vi "HandleObservationSync_003.vi"(8 "error in (no error)":errorcluster, 11 "S4GUI in":refnum<class "S4GUI.lvclass">) -> (0 "error out":errorcluster, 3 "S4GUI out":refnum<class "S4GUI.lvclass">)   [LabVIEW 2018, in "S4GUI.lvclass"] (continued)
          n1020 = call-dynamic "Write AcquisitionD.vi"("error in (no error)"=w2625, "Acquisition.lvclass"=w2621, "S4ACS_GUI in"=w2622) -> ("error out"=w2620:errorcluster, "S4ACS_GUI out"=w2619:refnum<class "S4GUI.lvclass">)  [unwired: 7 in]
          n1021 = Compound Arithmetic op=ADD(w2607, w2606, w2605, w2604) -> (w2608:u32)
          n1022 = case shown="0, Default" w2608 {
            tunnel: w2603 -> [w2645 _ _ _ _ _ _ _ _ _ _ _ _ _ _ _]
            tunnel: [w2644 u32 1 ("Obs_state") u32 1 ("Obs_state") u32 1 ("Obs_state") u32 1 ("Obs_state") u32 1 ("Obs_state") u32 1 ("Obs_state") u32 1 ("Obs_state") u32 1 ("Obs_state") u32 1 ("Obs_state") u32 1 ("Obs_state") u32 1 ("Obs_state") u32 1 ("Obs_state") u32 1 ("Obs_state") u32 1 ("Obs_state") u32 1 ("Obs_state")] -> w2609
            tunnel: ["" ("Error Msg") "ERROR: Lost channel 1 connection... - HandleObservationSync.vi state 308" ("Error Msg") "ERROR: Lost channel 2 connection...- HandleObservationSync.vi state 308" ("Error Msg") "ERROR: Lost channels 1 and 2 connection...- HandleObservationSync.vi state 308" ("Error Msg") "ERROR: Lost channel 3 connection...- HandleObservationSync.vi state 308" ("Error Msg") "ERROR: Lost channels 1 and  3 connection...- HandleObservationSync.vi state 308" ("Error Msg") "ERROR:  Lost channels 2 and  3 connection...- HandleObservationSync.vi state 308" ("Error Msg") "ERROR:  Lost channels 1, 2 and  3 connection...- HandleObservationSync.vi state 308" ("Error Msg") "ERROR: Lost channel 4 connection...- HandleObservationSync.vi state 308" ("Error Msg") "ERROR:  Lost channels 1 and 4 connection...- HandleObservationSync.vi state 308" ("Error Msg") "ERROR:  Lost channels 2 and 4 connection...- HandleObservationSync.vi state 308" ("Error Msg") "ERROR: Lost channels 1, 2 and 4 connection...- HandleObservationSync.vi state 308" ("Error Msg") "ERROR: Lost channels 3 and 4 connection...- HandleObservationSync.vi state 308" ("Error Msg") "ERROR: Lost channels 1, 3 and 4 connection...- HandleObservationSync.vi state 308" ("Error Msg") "ERROR: Lost channels 2, 3 and 4 connection...- HandleObservationSync.vi state 308" ("Error Msg") "ERROR: Lost channels 1, 2, 3 and 4 connection...- HandleObservationSync.vi state 308" ("Error Msg")] -> w2610
            frame 0, Default {
              n1023 = Tick Count (ms)() -> (millisecond timer value=w2642:u32)
              n1024 = Increment(x=w2645) -> (x+1=w2644:u32)
              n1025 = local write "time1"(w2642) -> ()
            }
            frame 1 {
            }
            frame 2 {
            }
            frame 3 {
            }
            frame 4 {
            }
            frame 5 {
            }
            frame 6 {
            }
            frame 7 {
            }
            frame 8 {
            }
            frame 9 {
            }
            frame 10 {
            }
            frame 11 {
            }
            frame 12 {
            }
            frame 13 {
            }
            frame 14 {
            }
            frame 15 {
            }
          }
          n1026 = Bundle By Name(cluster=w2619, "Obs_state"=w2609, "Error Msg"=w2610) -> (w2636:refnum<class "S4GUI.lvclass">)
        }
        frame 309 {
          # "Se wait_expose=T, não envia\no EXPOSE do estado 310\n(1o EXPOSE já foi enviado).\n\nNeste caso, vai para:\n* 310 se houver mais \n   de 1 posição da lamina ou para \n* 327 se houver apenas 1 posição\n   da lâmina"
          # "T: mode EXPOSE\nF: mode FIRE"
          # "Espera todos os canais chegarem ao estado ACTIVE\n(estados 54 e 55 de Channel:Run.vi)\n   OU\nTodos os canais incrementarem o Seqs_done. (OV 20240821)"
          n1027 = Unbundle By Name(w2770) -> ("seqAtual"=w2769:u32)
          n1028 = call-dynamic "Read AcquisitionA.vi"("error in (no error)"=w2830, "S4ACS_GUI in"=w2770) -> ("error out"=w2810:errorcluster, "Acquisition.lvclass"=w2811:refnum<class "Acquisition.lvclass">, "S4ACS_GUI out"=w2832:refnum<class "S4GUI.lvclass">)  [unwired: 7 in]
          n1029 = call "Read connection.vi"("error in (no error)"=w2810, "Server in"=w2811) -> ("error out"=w2812:errorcluster, "connection"=w2814:bool, "Server out"=w2813:refnum<class "Acquisition.lvclass">)  [unwired: 7 in]
          n1030 = case shown="True" w2814 {
            tunnel: [w2979 w3003] -> w2833
            tunnel: [w2978 w3002] -> w2831
            tunnel: w2813 -> [w2979 w2995]
            tunnel: w2812 -> [w2978 w2994]
            tunnel: [TRUE w2993] -> w2793
            tunnel: [FALSE w2987] -> w2789
            tunnel: [TRUE w2981] -> w2774
            tunnel: w2769 -> [_ w2980]
            frame False {
            }
            frame True {
              n1031 = call-dynamic "Read Channel.vi"("error in (no error)"=w2994, "Acquisition in"=w2995) -> ("error out"=w2984:errorcluster, "Channel.lvclass"=w2986:refnum<class "Channel.lvclass">, "Acquisition out"=w3004:refnum<class "Acquisition.lvclass">)  [unwired: 7 in]
              n1032 = call-dynamic "Read SequesDone.vi"("error in (no error)"=w2984, "Channel in"=w2986) -> ("error out"=w2983:errorcluster, "SequesDoneRaw"=w2982:u32, "Channel out"=w2985:refnum<class "Channel.lvclass">)  [unwired: 6 in, 1 out]
              n1033 = Equal?(x=w2982, y=w2980) -> (x = y?=w2981:bool)
              n1034 = call-dynamic "Read wait_expose.vi"("error in (no error)"=w2983, "Channel in"=w2985) -> ("error out"=w2988:errorcluster, "wait_expose"=w2987:bool, "Channel out"=w2989:refnum<class "Channel.lvclass">)  [unwired: 7 in]
              n1035 = call-dynamic "Read State Machine.vi"("error in (no error)"=w2988, "Device in"=w2989) -> ("error out"=w2996:errorcluster, "State Machine.lvclass"=w2998:refnum<class "State Machine.lvclass">, "Device out"=w3000:refnum<class "Channel.lvclass">)  [unwired: 7 in]
              n1036 = call-dynamic "Read State.vi"("error in (no error)"=w2996, "State Machine in"=w2998) -> ("error out"=w2990:errorcluster, "State"=w2992:i32, "State Machine out"=w2997:refnum<class "State Machine.lvclass">)  [unwired: 7 in]
              n1037 = Greater?(x=w2992, y=53) -> (0:w2993:bool)
              n1038 = call-dynamic "Write State Machine.vi"("error in (no error)"=w2990, "State Machine.lvclass"=w2997, "Device in"=w3000) -> ("error out"=w2999:errorcluster, "Device out"=w3001:refnum<class "Channel.lvclass">)  [unwired: 7 in]
              n1039 = call-dynamic "Write Channel.vi"("error in (no error)"=w2999, "Channel.lvclass"=w3001, "Acquisition in"=w3004) -> ("error out"=w3002:errorcluster, "Acquisition out"=w3003:refnum<class "Acquisition.lvclass">)  [unwired: 7 in]
            }
          }
          n1040 = call-dynamic "Write AcquisitionA.vi"("error in (no error)"=w2831, "Acquisition.lvclass"=w2833, "S4ACS_GUI in"=w2832) -> ("error out"=w2827:errorcluster, "S4ACS_GUI out"=w2828:refnum<class "S4GUI.lvclass">)  [unwired: 7 in]
          n1041 = call "Read AcquisitionB.vi"("error in (no error)"=w2827, "S4ACS_GUI in"=w2828) -> ("error out"=w2807:errorcluster, "Acquisition.lvclass"=w2809:refnum<class "Acquisition.lvclass">, "S4ACS_GUI out"=w2825:refnum<class "S4GUI.lvclass">)  [unwired: 7 in]
          n1042 = call "Read connection.vi"("error in (no error)"=w2807, "Server in"=w2809) -> ("error out"=w2806:errorcluster, "connection"=w2805:bool, "Server out"=w2808:refnum<class "Acquisition.lvclass">)  [unwired: 7 in]
          n1043 = case shown="True" w2805 {
            tunnel: w2808 -> [w2949 w2974]
            tunnel: w2806 -> [w2948 w2973]
            tunnel: [w2949 w2971] -> w2826
            tunnel: [w2948 w2970] -> w2824
            tunnel: [TRUE w2961] -> w2792
            tunnel: [FALSE ("expose") w2957] -> w2788
            tunnel: [TRUE w2951] -> w2776
            tunnel: w2769 -> [_ w2950]
            frame False {
            }
            frame True {
              n1044 = call-dynamic "Read Channel.vi"("error in (no error)"=w2973, "Acquisition in"=w2974) -> ("error out"=w2953:errorcluster, "Channel.lvclass"=w2956:refnum<class "Channel.lvclass">, "Acquisition out"=w2972:refnum<class "Acquisition.lvclass">)  [unwired: 7 in]
              n1045 = call-dynamic "Read SequesDone.vi"("error in (no error)"=w2953, "Channel in"=w2956) -> ("error out"=w2952:errorcluster, "SequesDoneRaw"=w2954:u32, "Channel out"=w2955:refnum<class "Channel.lvclass">)  [unwired: 6 in, 1 out]
              n1046 = Equal?(x=w2954, y=w2950) -> (x = y?=w2951:bool)
              n1047 = call-dynamic "Read wait_expose.vi"("error in (no error)"=w2952, "Channel in"=w2955) -> ("error out"=w2958:errorcluster, "wait_expose"=w2957:bool, "Channel out"=w2959:refnum<class "Channel.lvclass">)  [unwired: 7 in]
              n1048 = call-dynamic "Read State Machine.vi"("error in (no error)"=w2958, "Device in"=w2959) -> ("error out"=w2964:errorcluster, "State Machine.lvclass"=w2966:refnum<class "State Machine.lvclass">, "Device out"=w2968:refnum<class "Channel.lvclass">)  [unwired: 7 in]
              n1049 = call-dynamic "Read State.vi"("error in (no error)"=w2964, "State Machine in"=w2966) -> ("error out"=w2963:errorcluster, "State"=w2960:i32, "State Machine out"=w2965:refnum<class "State Machine.lvclass">)  [unwired: 7 in]
              n1050 = Greater?(x=w2960, y=53) -> (0:w2961:bool)
              n1051 = call-dynamic "Write State Machine.vi"("error in (no error)"=w2963, "State Machine.lvclass"=w2965, "Device in"=w2968) -> ("error out"=w2967:errorcluster, "Device out"=w2969:refnum<class "Channel.lvclass">)  [unwired: 7 in]
              n1052 = call-dynamic "Write Channel.vi"("error in (no error)"=w2967, "Channel.lvclass"=w2969, "Acquisition in"=w2972) -> ("error out"=w2970:errorcluster, "Acquisition out"=w2971:refnum<class "Acquisition.lvclass">)  [unwired: 7 in]
            }
          }
          n1053 = call "Write AcquisitionB.vi"("error in (no error)"=w2824, "Acquisition.lvclass"=w2826, "S4ACS_GUI in"=w2825) -> ("error out"=w2820:errorcluster, "S4ACS_GUI out"=w2819:refnum<class "S4GUI.lvclass">)  [unwired: 7 in]
          n1054 = call-dynamic "Read AcquisitionC.vi"("error in (no error)"=w2820, "S4ACS_GUI in"=w2819) -> ("error out"=w2802:errorcluster, "Acquisition.lvclass"=w2804:refnum<class "Acquisition.lvclass">, "S4ACS_GUI out"=w2822:refnum<class "S4GUI.lvclass">)  [unwired: 7 in]
          n1055 = call "Read connection.vi"("error in (no error)"=w2802, "Server in"=w2804) -> ("error out"=w2801:errorcluster, "connection"=w2800:bool, "Server out"=w2803:refnum<class "Acquisition.lvclass">)  [unwired: 7 in]
          n1056 = case shown="True" w2800 {
            tunnel: [w2918 w2939] -> w2823
            tunnel: [w2919 w2938] -> w2821
            tunnel: w2803 -> [w2919 w2934]
            tunnel: w2801 -> [w2918 w2933]
            tunnel: [TRUE w2930] -> w2791
            tunnel: [FALSE ("expose") w2927] -> w2787
            tunnel: [TRUE w2921] -> w2775
            tunnel: w2769 -> [_ w2920]
            frame False {
            }
            frame True {
              n1057 = call-dynamic "Read Channel.vi"("error in (no error)"=w2933, "Acquisition in"=w2934) -> ("error out"=w2926:errorcluster, "Channel.lvclass"=w2925:refnum<class "Channel.lvclass">, "Acquisition out"=w2937:refnum<class "Acquisition.lvclass">)  [unwired: 7 in]
              n1058 = call-dynamic "Read SequesDone.vi"("error in (no error)"=w2926, "Channel in"=w2925) -> ("error out"=w2922:errorcluster, "SequesDoneRaw"=w2923:u32, "Channel out"=w2924:refnum<class "Channel.lvclass">)  [unwired: 6 in, 1 out]
              n1059 = Equal?(x=w2923, y=w2920) -> (x = y?=w2921:bool)
              n1060 = call-dynamic "Read wait_expose.vi"("error in (no error)"=w2922, "Channel in"=w2924) -> ("error out"=w2928:errorcluster, "wait_expose"=w2927:bool, "Channel out"=w2929:refnum<class "Channel.lvclass">)  [unwired: 7 in]
              n1061 = call-dynamic "Read State Machine.vi"("error in (no error)"=w2928, "Device in"=w2929) -> ("error out"=w2935:errorcluster, "State Machine.lvclass"=w2943:refnum<class "State Machine.lvclass">, "Device out"=w2941:refnum<class "Channel.lvclass">)  [unwired: 7 in]
              n1062 = call-dynamic "Read State.vi"("error in (no error)"=w2935, "State Machine in"=w2943) -> ("error out"=w2936:errorcluster, "State"=w2931:i32, "State Machine out"=w2944:refnum<class "State Machine.lvclass">)  [unwired: 7 in]
              n1063 = Greater?(x=w2931, y=53) -> (0:w2930:bool)
              n1064 = call-dynamic "Write State Machine.vi"("error in (no error)"=w2936, "State Machine.lvclass"=w2944, "Device in"=w2941) -> ("error out"=w2942:errorcluster, "Device out"=w2940:refnum<class "Channel.lvclass">)  [unwired: 7 in]
              n1065 = call-dynamic "Write Channel.vi"("error in (no error)"=w2942, "Channel.lvclass"=w2940, "Acquisition in"=w2937) -> ("error out"=w2939:errorcluster, "Acquisition out"=w2938:refnum<class "Acquisition.lvclass">)  [unwired: 7 in]
            }
          }
          n1066 = call-dynamic "Write AcquisitionC.vi"("error in (no error)"=w2823, "Acquisition.lvclass"=w2821, "S4ACS_GUI in"=w2822) -> ("error out"=w2799:errorcluster, "S4ACS_GUI out"=w2815:refnum<class "S4GUI.lvclass">)  [unwired: 7 in]
          n1067 = call-dynamic "Read AcquisitionD.vi"("error in (no error)"=w2799, "S4ACS_GUI in"=w2815) -> ("error out"=w2795:errorcluster, "Acquisition.lvclass"=w2798:refnum<class "Acquisition.lvclass">, "S4ACS_GUI out"=w2817:refnum<class "S4GUI.lvclass">)  [unwired: 7 in]
          n1068 = call "Read connection.vi"("error in (no error)"=w2795, "Server in"=w2798) -> ("error out"=w2796:errorcluster, "connection"=w2794:bool, "Server out"=w2797:refnum<class "Acquisition.lvclass">)  [unwired: 7 in]
          n1069 = case shown="True" w2794 {
            tunnel: [w2889 w2913] -> w2818
            tunnel: [w2888 w2912] -> w2816
            tunnel: [TRUE w2901] -> w2790
            tunnel: w2797 -> [w2889 w2904]
            tunnel: w2796 -> [w2888 w2903]
            tunnel: [FALSE ("expose") w2897] -> w2786
            tunnel: [TRUE w2891] -> w2777
            tunnel: w2769 -> [_ w2890]
            frame False {
            }
            frame True {
              n1070 = call-dynamic "Read Channel.vi"("error in (no error)"=w2903, "Acquisition in"=w2904) -> ("error out"=w2895:errorcluster, "Channel.lvclass"=w2896:refnum<class "Channel.lvclass">, "Acquisition out"=w2914:refnum<class "Acquisition.lvclass">)  [unwired: 7 in]
              n1071 = call-dynamic "Read SequesDone.vi"("error in (no error)"=w2895, "Channel in"=w2896) -> ("error out"=w2893:errorcluster, "SequesDoneRaw"=w2894:u32, "Channel out"=w2892:refnum<class "Channel.lvclass">)  [unwired: 6 in, 1 out]
              n1072 = Equal?(x=w2894, y=w2890) -> (x = y?=w2891:bool)
              n1073 = call-dynamic "Read wait_expose.vi"("error in (no error)"=w2893, "Channel in"=w2892) -> ("error out"=w2898:errorcluster, "wait_expose"=w2897:bool, "Channel out"=w2899:refnum<class "Channel.lvclass">)  [unwired: 7 in]
              n1074 = call-dynamic "Read State Machine.vi"("error in (no error)"=w2898, "Device in"=w2899) -> ("error out"=w2906:errorcluster, "State Machine.lvclass"=w2908:refnum<class "State Machine.lvclass">, "Device out"=w2910:refnum<class "Channel.lvclass">)  [unwired: 7 in]
              n1075 = call-dynamic "Read State.vi"("error in (no error)"=w2906, "State Machine in"=w2908) -> ("error out"=w2905:errorcluster, "State"=w2900:i32, "State Machine out"=w2907:refnum<class "State Machine.lvclass">)  [unwired: 7 in]
              n1076 = Greater?(x=w2900, y=53) -> (0:w2901:bool)
              n1077 = call-dynamic "Write State Machine.vi"("error in (no error)"=w2905, "State Machine.lvclass"=w2907, "Device in"=w2910) -> ("error out"=w2909:errorcluster, "Device out"=w2911:refnum<class "Channel.lvclass">)  [unwired: 7 in]
              n1078 = call-dynamic "Write Channel.vi"("error in (no error)"=w2909, "Channel.lvclass"=w2911, "Acquisition in"=w2914) -> ("error out"=w2912:errorcluster, "Acquisition out"=w2913:refnum<class "Acquisition.lvclass">)  [unwired: 7 in]
            }
          }
          n1079 = call-dynamic "Write AcquisitionD.vi"("error in (no error)"=w2816, "Acquisition.lvclass"=w2818, "S4ACS_GUI in"=w2817) -> ("error out"=w2768:errorcluster, "S4ACS_GUI out"=w2766:refnum<class "S4GUI.lvclass">)  [unwired: 7 in]
          n1080 = Compound Arithmetic op=OR(w2789, w2788, w2787, w2786) -> (w2779:bool)
          n1081 = Compound Arithmetic op=AND(w2774, w2776, w2775, w2777) -> (w2772:bool)
          n1082 = Compound Arithmetic op=AND(w2793, w2792, w2791, w2790) -> (w2773:bool)
          n1083 = Or(x=w2773, y=w2772) -> (x .or. y?=w2771:bool)
          n1084 = call-dynamic "VerifErrors.vi"("error in (no error)"=w2768, "S4GUI in"=w2766) -> ("error out"=w2767:errorcluster, "Error value"=w2764:u32, "S4GUI out"=w2765:refnum<class "S4GUI.lvclass">)  [unwired: 7 in]
          n1085 = call-dynamic "VerifWavePlate.vi"("error in (no error)"=w2767, "S4GUI in"=w2765) -> ("error out"=w2783:errorcluster, "One Position"=w2785:bool, "S4GUI out"=w2784:refnum<class "S4GUI.lvclass">)  [unwired: 7 in]
          n1086 = case shown="True" w2785 {
            tunnel: w2784 -> [w2866 w2883]
            tunnel: [u32 312 ("t") u32 327 ("t")] -> w2781
            tunnel: [w2866 w2869] -> w2780
            tunnel: w2783 -> [w2864 w2868]
            tunnel: [w2864 w2867] -> w2782
            frame False {
            }
            frame True {
              # "Recarrega SEQ, antes de desviar\n para tratamento de fotometria."
              n1087 = call "Read Instrument.lvclass.vi"("error in (no error)"=w2868, "S4ACS_GUI in"=w2883) -> ("error out"=w2878:errorcluster, "Instrument.lvclass"=w2882:refnum<class "Instrument.lvclass">, "S4ACS_GUI out"=w2881:refnum<class "S4GUI.lvclass">)  [unwired: 7 in]
              n1088 = call "Read WPROT.vi"("error in (no error)"=w2878, "Instrument in"=w2882) -> ("error out"=w2871:errorcluster, "Opt_Selector.lvclass"=w2874:refnum<class "Opt_Selector.lvclass">, "Instrument out"=w2879:refnum<class "Instrument.lvclass">)  [unwired: 7 in]
              n1089 = call-dynamic "Read sequencia_ant.vi"("error in (no error)"=w2871, "Opt_Selector in"=w2874) -> ("error out"=w2876:errorcluster, "sequencia_ant"=w2875:u16, "Opt_Selector out"=w2873:refnum<class "Opt_Selector.lvclass">)  [unwired: 7 in]
              n1090 = call-dynamic "Write sequencia.vi"("error in (no error)"=w2876, "sequencia"=w2875, "Opt_Selector in"=w2873) -> ("error out"=w2870:errorcluster, "Opt_Selector out"=w2872:refnum<class "Opt_Selector.lvclass">)  [unwired: 7 in]
              n1091 = call "Write WPROT.vi"("error in (no error)"=w2870, "Opt_Selector.lvclass"=w2872, "Instrument in"=w2879) -> ("error out"=w2877:errorcluster, "Instrument out"=w2880:refnum<class "Instrument.lvclass">)  [unwired: 7 in]
              n1092 = call "Write Instrument.lvclass.vi"("error in (no error)"=w2877, "Instrument.lvclass"=w2880, "S4ACS_GUI in"=w2881) -> ("error out"=w2867:errorcluster, "S4ACS_GUI out"=w2869:refnum<class "S4GUI.lvclass">)  [unwired: 7 in]
            }
          }
          n1093 = case shown="False" w2771 {
            tunnel: w2780 -> [w2836 w2863]
            tunnel: [w2842 w2862] -> w2778
            tunnel: w2781 -> [_ w2860]
            tunnel: w2764 -> [w2834 _]
            frame False {
              # "Aguardando iniciar exposição por 5s"
              n1094 = Tick Count (ms)() -> (millisecond timer value=w2841:u32)
              n1095 = local read "time1"() -> (w2835:u32)
              n1096 = Subtract(x=w2841, y=w2835) -> (x-y=w2838:u32)
              n1097 = To Double Precision Float(number=w2838) -> (double precision float=w2840:dbl)
              n1098 = Less?(x=5000.0 ("y"), y=w2840) -> (x < y?=w2839:bool)
              n1099 = case shown="False" w2839 {
                tunnel: w2836 -> [w2844 w2858]
                tunnel: [w2843 w2857] -> w2842
                tunnel: w2834 -> [w2845 _]
                frame False {
                  n1100 = case shown="1..15" w2845 {
                    selector: w2845 -> [_ w2853]
                    tunnel: [w2846 w2848] -> w2843
                    tunnel: w2844 -> [w2846 w2854]
                    frame 0, Default {
                    }
                    frame 1..15 {
                      n1101 = Number To Decimal String(number=w2853) -> (decimal integer string=w2850:string)  [unwired: 1 in]
                      n1102 = Concatenate Strings("CHANNEL ERROR <", w2850, ">: Error flag TRUE - see ACS panel.  HandleObservationSync.vi - state 309.") -> (w2852:string)
                      n1103 = Bundle By Name(cluster=w2854, "Obs_state"=u32 1, "Error Msg"=w2852) -> (w2848:refnum<class "S4GUI.lvclass">)
                    }
                  }
                }
                frame True {
                  n1104 = Bundle By Name(cluster=w2858, "Obs_state"=u32 1, "Error Msg"="ERROR: Acquisition Timeout. HandleObservationSync.vi - state 309.") -> (w2857:refnum<class "S4GUI.lvclass">)
                }
              }
            }
            frame True {
              # "Iniciou aquisição..."
              n1105 = Tick Count (ms)() -> (millisecond timer value=→"time308":u32)
              n1106 = Tick Count (ms)() -> (millisecond timer value=w2861:u32)
              n1107 = Bundle By Name(cluster=w2863, "Obs_state"=w2860) -> (w2862:refnum<class "S4GUI.lvclass">)
              n1108 = local write "time307"(w2861) -> ()
              n1109 = local write "time1"(w2861) -> ()
            }
          }
          n1110 = Bundle By Name(cluster=w2778, "mode EXPOSE"=w2779) -> (w2829:refnum<class "S4GUI.lvclass">)
        }
        frame 312 {
          # "Verifcando avanço de SEQUENCIA:"
          # "T=canais receberam STOP"
          # "T= Todos os canais ativos na mesma sequencia;\nF= Canais com sequencia diferente"
          # "Todos os SEQ_DONE \nsão iguais a SeqAtual?\nSe sim, avança lâmina."
          # "Exemplo:\nSET #CYCLES 3\nSET #SEQ 4\ntotal de sequencias: 3 x 4 = 12\n\nseq.        CYCLES_DONE           SEQS_DONE\n1a.                     0                                 0\n2a.                     0                                 1 \n3a.                     0                                 2 \n4a.                     0                                 3 \n                          1                                 4\n5a.                     1                                 0 \n6a.                     1                                 1 \n7a.                     1                                 2 \n8a.                     1                                 3 \n                          2                                 4\n9a.                     2                                 0 \n10a.                   2                                 1 \n11a.                   2                                 2 \n12a.                   2                                 3 \n\nfim                    3                                 4"
          n1111 = Unbundle By Name(w3030) -> ("seqAtual"=w3027:u32)
          n1112 = call-dynamic "Read AcquisitionA.vi"("error in (no error)"=w3064, "S4ACS_GUI in"=w3030) -> ("error out"=w3045:errorcluster, "Acquisition.lvclass"=w3046:refnum<class "Acquisition.lvclass">, "S4ACS_GUI out"=w3066:refnum<class "S4GUI.lvclass">)  [unwired: 7 in]
          n1113 = call-dynamic "Read enabled.vi"("error in (no error)"=w3045, "Server in"=w3046) -> ("error out"=w3044:errorcluster, "enabled"=w3019:bool, "Server out"=w3043:refnum<class "Acquisition.lvclass">)  [unwired: 7 in]
          n1114 = case shown="True" w3019 {
            tunnel: w3044 -> [w3215 w3231]
            tunnel: [w3216 w3229] -> w3067
            tunnel: [w3215 w3228] -> w3065
            tunnel: [u32 0 ("SequesDone") w3217] -> w3024
            tunnel: w3043 -> [w3216 w3227]
            tunnel: w3027 -> [_ w3226]
            tunnel: [TRUE w3225] -> w3029
            tunnel: [FALSE ("stopping") w3218] -> w3012
            frame False {
            }
            frame True {
              # "SEQS_DONE = 0,1,2,...,n,0,1,..."
              n1115 = call-dynamic "Read Channel.vi"("error in (no error)"=w3231, "Acquisition in"=w3227) -> ("error out"=w3223:errorcluster, "Channel.lvclass"=w3224:refnum<class "Channel.lvclass">, "Acquisition out"=w3230:refnum<class "Acquisition.lvclass">)  [unwired: 7 in]
              n1116 = call-dynamic "Read SequesDone.vi"("error in (no error)"=w3223, "Channel in"=w3224) -> ("error out"=w3221:errorcluster, "SequesDoneRaw"=w3217:u32, "Channel out"=w3222:refnum<class "Channel.lvclass">)  [unwired: 6 in, 1 out]
              n1117 = Equal?(x=w3217, y=w3226) -> (x = y?=w3225:bool)
              n1118 = call-dynamic "Read stopping.vi"("error in (no error)"=w3221, "Channel in"=w3222) -> ("error out"=w3220:errorcluster, "stopping"=w3218:bool, "Channel out"=w3219:refnum<class "Channel.lvclass">)  [unwired: 7 in]
              n1119 = call-dynamic "Write Channel.vi"("error in (no error)"=w3220, "Channel.lvclass"=w3219, "Acquisition in"=w3230) -> ("error out"=w3228:errorcluster, "Acquisition out"=w3229:refnum<class "Acquisition.lvclass">)  [unwired: 7 in]
            }
          }
          n1120 = call-dynamic "Write AcquisitionA.vi"("error in (no error)"=w3065, "Acquisition.lvclass"=w3067, "S4ACS_GUI in"=w3066) -> ("error out"=w3062:errorcluster, "S4ACS_GUI out"=w3061:refnum<class "S4GUI.lvclass">)  [unwired: 7 in]
          n1121 = call "Read AcquisitionB.vi"("error in (no error)"=w3062, "S4ACS_GUI in"=w3061) -> ("error out"=w3039:errorcluster, "Acquisition.lvclass"=w3042:refnum<class "Acquisition.lvclass">, "S4ACS_GUI out"=w3063:refnum<class "S4GUI.lvclass">)  [unwired: 7 in]
          n1122 = call-dynamic "Read enabled.vi"("error in (no error)"=w3039, "Server in"=w3042) -> ("error out"=w3040:errorcluster, "enabled"=w3018:bool, "Server out"=w3041:refnum<class "Acquisition.lvclass">)  [unwired: 7 in]
          n1123 = case shown="True" w3018 {
            tunnel: w3040 -> [w3195 w3211]
            tunnel: w3041 -> [w3196 w3210]
            tunnel: [u32 0 ("SequesDone") w3197] -> w3021
            tunnel: [w3195 w3209] -> w3060
            tunnel: [w3196 w3208] -> w3059
            tunnel: w3027 -> [_ w3205]
            tunnel: [TRUE w3204] -> w3028
            tunnel: [FALSE ("stopping") w3198] -> w3011
            frame False {
            }
            frame True {
              n1124 = call-dynamic "Read Channel.vi"("error in (no error)"=w3211, "Acquisition in"=w3210) -> ("error out"=w3202:errorcluster, "Channel.lvclass"=w3203:refnum<class "Channel.lvclass">, "Acquisition out"=w3206:refnum<class "Acquisition.lvclass">)  [unwired: 7 in]
              n1125 = call-dynamic "Read SequesDone.vi"("error in (no error)"=w3202, "Channel in"=w3203) -> ("error out"=w3200:errorcluster, "SequesDoneRaw"=w3197:u32, "Channel out"=w3207:refnum<class "Channel.lvclass">)  [unwired: 6 in, 1 out]
              n1126 = Equal?(x=w3197, y=w3205) -> (x = y?=w3204:bool)
              n1127 = call-dynamic "Read stopping.vi"("error in (no error)"=w3200, "Channel in"=w3207) -> ("error out"=w3199:errorcluster, "stopping"=w3198:bool, "Channel out"=w3201:refnum<class "Channel.lvclass">)  [unwired: 7 in]
              n1128 = call-dynamic "Write Channel.vi"("error in (no error)"=w3199, "Channel.lvclass"=w3201, "Acquisition in"=w3206) -> ("error out"=w3209:errorcluster, "Acquisition out"=w3208:refnum<class "Acquisition.lvclass">)  [unwired: 7 in]
            }
          }
          n1129 = call "Write AcquisitionB.vi"("error in (no error)"=w3060, "Acquisition.lvclass"=w3059, "S4ACS_GUI in"=w3063) -> ("error out"=w3052:errorcluster, "S4ACS_GUI out"=w3051:refnum<class "S4GUI.lvclass">)  [unwired: 7 in]
          n1130 = call-dynamic "Read AcquisitionC.vi"("error in (no error)"=w3052, "S4ACS_GUI in"=w3051) -> ("error out"=w3036:errorcluster, "Acquisition.lvclass"=w3038:refnum<class "Acquisition.lvclass">, "S4ACS_GUI out"=w3054:refnum<class "S4GUI.lvclass">)  [unwired: 7 in]
          n1131 = call-dynamic "Read enabled.vi"("error in (no error)"=w3036, "Server in"=w3038) -> ("error out"=w3035:errorcluster, "enabled"=w3017:bool, "Server out"=w3037:refnum<class "Acquisition.lvclass">)  [unwired: 7 in]
          n1132 = case shown="True" w3017 {
            tunnel: [w3175 w3191] -> w3055
            tunnel: [w3176 w3190] -> w3053
            tunnel: w3035 -> [w3175 w3187]
            tunnel: w3037 -> [w3176 w3188]
            tunnel: [u32 0 ("SequesDone") w3177] -> w3020
            tunnel: w3027 -> [_ w3186]
            tunnel: [TRUE w3185] -> w3026
            tunnel: [FALSE ("stopping") w3178] -> w3010
            frame False {
            }
            frame True {
              n1133 = call-dynamic "Read Channel.vi"("error in (no error)"=w3187, "Acquisition in"=w3188) -> ("error out"=w3182:errorcluster, "Channel.lvclass"=w3183:refnum<class "Channel.lvclass">, "Acquisition out"=w3189:refnum<class "Acquisition.lvclass">)  [unwired: 7 in]
              n1134 = call-dynamic "Read SequesDone.vi"("error in (no error)"=w3182, "Channel in"=w3183) -> ("error out"=w3180:errorcluster, "SequesDoneRaw"=w3177:u32, "Channel out"=w3184:refnum<class "Channel.lvclass">)  [unwired: 6 in, 1 out]
              n1135 = Equal?(x=w3177, y=w3186) -> (x = y?=w3185:bool)
              n1136 = call-dynamic "Read stopping.vi"("error in (no error)"=w3180, "Channel in"=w3184) -> ("error out"=w3179:errorcluster, "stopping"=w3178:bool, "Channel out"=w3181:refnum<class "Channel.lvclass">)  [unwired: 7 in]
              n1137 = call-dynamic "Write Channel.vi"("error in (no error)"=w3179, "Channel.lvclass"=w3181, "Acquisition in"=w3189) -> ("error out"=w3191:errorcluster, "Acquisition out"=w3190:refnum<class "Acquisition.lvclass">)  [unwired: 7 in]
            }
          }
          n1138 = call-dynamic "Write AcquisitionC.vi"("error in (no error)"=w3055, "Acquisition.lvclass"=w3053, "S4ACS_GUI in"=w3054) -> ("error out"=w3049:errorcluster, "S4ACS_GUI out"=w3050:refnum<class "S4GUI.lvclass">)  [unwired: 7 in]
          n1139 = call-dynamic "Read AcquisitionD.vi"("error in (no error)"=w3049, "S4ACS_GUI in"=w3050) -> ("error out"=w3032:errorcluster, "Acquisition.lvclass"=w3034:refnum<class "Acquisition.lvclass">, "S4ACS_GUI out"=w3056:refnum<class "S4GUI.lvclass">)  [unwired: 7 in]
          n1140 = call-dynamic "Read enabled.vi"("error in (no error)"=w3032, "Server in"=w3034) -> ("error out"=w3031:errorcluster, "enabled"=w3016:bool, "Server out"=w3033:refnum<class "Acquisition.lvclass">)  [unwired: 7 in]
          n1141 = Build Array(w3019, w3018, w3017, w3016) -> (w3015:bool[])
          n1142 = case shown="True" w3016 {
            tunnel: [w3156 w3171] -> w3058
            tunnel: [w3155 w3170] -> w3057
            tunnel: w3033 -> [w3156 w3169]
            tunnel: w3031 -> [w3155 w3168]
            tunnel: [u32 0 ("SequesDone") w3157] -> w3023
            tunnel: w3027 -> [_ w3166]
            tunnel: [TRUE w3165] -> w3025
            tunnel: [FALSE ("stopping") w3158] -> w3009
            frame False {
            }
            frame True {
              n1143 = call-dynamic "Read Channel.vi"("error in (no error)"=w3168, "Acquisition in"=w3169) -> ("error out"=w3162:errorcluster, "Channel.lvclass"=w3163:refnum<class "Channel.lvclass">, "Acquisition out"=w3167:refnum<class "Acquisition.lvclass">)  [unwired: 7 in]
              n1144 = call-dynamic "Read SequesDone.vi"("error in (no error)"=w3162, "Channel in"=w3163) -> ("error out"=w3160:errorcluster, "SequesDoneRaw"=w3157:u32, "Channel out"=w3164:refnum<class "Channel.lvclass">)  [unwired: 6 in, 1 out]
              n1145 = Equal?(x=w3157, y=w3166) -> (x = y?=w3165:bool)
              n1146 = call-dynamic "Read stopping.vi"("error in (no error)"=w3160, "Channel in"=w3164) -> ("error out"=w3159:errorcluster, "stopping"=w3158:bool, "Channel out"=w3161:refnum<class "Channel.lvclass">)  [unwired: 7 in]
              n1147 = call-dynamic "Write Channel.vi"("error in (no error)"=w3159, "Channel.lvclass"=w3161, "Acquisition in"=w3167) -> ("error out"=w3170:errorcluster, "Acquisition out"=w3171:refnum<class "Acquisition.lvclass">)  [unwired: 7 in]
            }
          }
          n1148 = Boolean Array To Number(Boolean array=w3015) -> (number=w3013:u32)
          n1149 = Compound Arithmetic op=AND(w3029, w3028, w3026, w3025) -> (w3014:bool)
          n1150 = Compound Arithmetic op=OR(w3012, w3011, w3010, w3009) -> (w3008:bool)
          n1151 = case shown="11" w3013 {
            tunnel: w3024 -> [w3075 _ w3087 _ w3096 _ w3102 w3108 _ w3114 w3117 _]
            tunnel: w3023 -> [w3074 w3078 w3083 w3090 w3091 w3099 w3101 _ _ _ _ _]
            tunnel: w3021 -> [w3073 w3076 _ _ w3095 w3097 _ w3107 w3111 _ w3116 _]
            tunnel: w3020 -> [w3072 w3077 w3082 w3088 _ _ _ w3106 w3110 w3113 _ _]
            tunnel: [w3068 w3079 w3084 w3089 w3092 w3098 w3100 w3103 w3109 w3112 w3115 TRUE] -> _
            frame 15 {
              # "A,B,C,D ativos"
              n1152 = Equal?(x=w3075, y=w3073) -> (x = y?=w3071:bool)
              n1153 = Equal?(x=w3072, y=w3074) -> (x = y?=w3069:bool)
              n1154 = Equal?(x=w3073, y=w3072) -> (x = y?=w3070:bool)
              n1155 = Compound Arithmetic op=AND(w3071, w3070, w3069) -> (w3068:bool)
            }
            frame 14 {
              # "B,C e,D ativos"
              n1156 = Equal?(x=w3076, y=w3077) -> (x = y?=w3081:bool)
              n1157 = Equal?(x=w3077, y=w3078) -> (x = y?=w3080:bool)
              n1158 = Compound Arithmetic op=AND(w3081, w3080) -> (w3079:bool)
            }
            frame 13 {
              # "A,C e,D ativos"
              n1159 = Equal?(x=w3087, y=w3082) -> (x = y?=w3086:bool)
              n1160 = Equal?(x=w3082, y=w3083) -> (x = y?=w3085:bool)
              n1161 = Compound Arithmetic op=AND(w3086, w3085) -> (w3084:bool)
            }
            frame 12 {
              # "Só C e D ativos"
              n1162 = Equal?(x=w3088, y=w3090) -> (x = y?=w3089:bool)
            }
            frame 11 {
              # "A,B e,D ativos"
              n1163 = Equal?(x=w3096, y=w3095) -> (x = y?=w3094:bool)
              n1164 = Equal?(x=w3095, y=w3091) -> (x = y?=w3093:bool)
              n1165 = Compound Arithmetic op=AND(w3094, w3093) -> (w3092:bool)
            }
            frame 10 {
              # "Só B e D ativos"
              n1166 = Equal?(x=w3097, y=w3099) -> (x = y?=w3098:bool)
            }
            frame 9 {
              # "Só A e D ativos"
              n1167 = Equal?(x=w3102, y=w3101) -> (x = y?=w3100:bool)
            }
            frame 7 {
              # "A,B,C ativos"
              n1168 = Equal?(x=w3108, y=w3107) -> (x = y?=w3105:bool)
              n1169 = Equal?(x=w3107, y=w3106) -> (x = y?=w3104:bool)
              n1170 = Compound Arithmetic op=AND(w3105, w3104) -> (w3103:bool)
            }
            frame 6 {
              # "Só B e C ativos"
              n1171 = Equal?(x=w3111, y=w3110) -> (x = y?=w3109:bool)
            }
            frame 5 {
              # "Só A e C ativos"
              n1172 = Equal?(x=w3114, y=w3113) -> (x = y?=w3112:bool)
            }
            frame 3 {
              # "só A e B ativos"
              n1173 = Equal?(x=w3117, y=w3116) -> (x = y?=w3115:bool)
            }
            frame 0..2, 4, 8, Default {
              # "nenhum ou só 1  \ncanal ativo."
            }
          }
          n1174 = call-dynamic "Write AcquisitionD.vi"("error in (no error)"=w3057, "Acquisition.lvclass"=w3058, "S4ACS_GUI in"=w3056) -> ("error out"=w3047:errorcluster, "S4ACS_GUI out"=w3048:refnum<class "S4GUI.lvclass">)  [unwired: 7 in]
          n1175 = And(x=w3014, y=TRUE) -> (x .and. y?=w3022:bool)
          n1176 = case shown="True" w3022 {
            tunnel: w3048 -> [w3120 w3149]
            tunnel: [w3119 w3148] -> w3007
            tunnel: w3014 -> [w3121 _]
            tunnel: w3008 -> [_ w3147]
            tunnel: w3006 -> [_ w3142]
            frame False {
              n1177 = case shown="False" w3121 {
                tunnel: w3120 -> [w3128 w3141]
                tunnel: [w3132 w3140] -> w3119
                frame False {
                  # "Esperando todos os canais habilitados mudarem de sequesDone.\nE verificando a maior duracao de cubo entre os canais."
                  n1178 = local read "time307"() -> (w3131:u32)
                  n1179 = Tick Count (ms)() -> (millisecond timer value=w3130:u32)
                  n1180 = Subtract(x=w3130, y=w3131) -> (x-y=w3125:u32)
                  n1181 = call-dynamic "GetGreatestCube.vi"("S4GUI in"=w3128) -> ("S4GUI out"=w3127:refnum<class "S4GUI.lvclass">, "greatest (ms)"=w3123:dbl)  [unwired: 8 in, 1 out]
                  n1182 = To Double Precision Float(number=w3125) -> (double precision float=w3129:dbl)
                  n1183 = Add(x=1000.0 ("y"), y=w3123) -> (x+y=w3122:dbl)
                  n1184 = Less?(x=w3122, y=w3129) -> (x < y?=w3126:bool)
                  n1185 = case shown="True" w3126 {
                    tunnel: w3127 -> [w3133 w3137]
                    tunnel: [w3133 w3136] -> w3132
                    frame False {
                    }
                    frame True {
                      n1186 = Bundle By Name(cluster=w3137, "Obs_state"=u32 1, "Error Msg"="ERROR: Acquisition Timeout - HandleObservationSync.vi - state 312.") -> (w3136:refnum<class "S4GUI.lvclass">)
                    }
                  }
                }
                frame True {
                  # "Nunca entra aqui!!"
                  n1187 = Bundle By Name(cluster=w3141, "Obs_state"=u32 1, "Error Msg"="ERROR: Sequence_done not equal in all active channels.") -> (w3140:refnum<class "S4GUI.lvclass">)
                }
              }
            }
            frame True {
              # "STOP?"
              n1188 = local read "time308"() -> (w3145:u32)
              n1189 = Tick Count (ms)() -> (millisecond timer value=w3146:u32)
              n1190 = Subtract(x=w3146, y=w3145) -> (x-y=→"delay Acq":u32)
              n1191 = case shown="False" w3147 {
                tunnel: w3142 -> [_ _]
                tunnel: [u32 303 u32 0] -> w3143
                frame False {
                }
                frame True {
                }
              }
              n1192 = Bundle By Name(cluster=w3149, "Obs_state"=w3143) -> (w3148:refnum<class "S4GUI.lvclass">)
            }
          }
        }
        frame 314 {
          n1193 = Unbundle By Name(w3235) -> ("cyclesDone"=w3233:u32)
          n1194 = Increment(x=w3233) -> (x+1=w3232:u32)
          n1195 = Bundle By Name(cluster=w3235, "cyclesDone"=w3232) -> (w3234:refnum<class "S4GUI.lvclass">)
          n1196 = Unbundle By Name(w3234) -> ("TotalCiclos"=w3242:u32, "cyclesDone"=w3241:u32)
          n1197 = Subtract(x=w3242, y=w3241) -> (x-y=w3240:u32)
          n1198 = Greater Than 0?(x=w3240) -> (x > 0?=w3239:bool)
          n1199 = Select(t=u32 303, s=w3239, f=u32 0) -> (s? t:f=w3238:u32)
          n1200 = Bundle By Name(cluster=w3234, "Obs_state"=w3238) -> (w3243:refnum<class "S4GUI.lvclass">)
        }
        frame 321 {
          n1201 = call-dynamic "Read AcquisitionA.vi"("error in (no error)"=w3307, "S4ACS_GUI in"=w3308) -> ("error out"=w3262:errorcluster, "Acquisition.lvclass"=w3263:refnum<class "Acquisition.lvclass">, "S4ACS_GUI out"=w3310:refnum<class "S4GUI.lvclass">)  [unwired: 7 in]
          n1202 = call-dynamic "Read enabled.vi"("error in (no error)"=w3262, "Server in"=w3263) -> ("error out"=w3261:errorcluster, "enabled"=w3248:bool, "Server out"=w3264:refnum<class "Acquisition.lvclass">)  [unwired: 7 in]
          n1203 = call "Read connection.vi"("error in (no error)"=w3261, "Server in"=w3264) -> ("error out"=w3287:errorcluster, "connection"=w3271:bool, "Server out"=w3288:refnum<class "Acquisition.lvclass">)  [unwired: 7 in]
          n1204 = And(x=w3271, y=w3248) -> (x .and. y?=w3272:bool)
          n1205 = case shown="True" w3272 {
            tunnel: w3288 -> [w3425 w3444]
            tunnel: w3287 -> [w3424 w3443]
            tunnel: [w3425 w3441] -> w3311
            tunnel: [w3424 w3440] -> w3309
            tunnel: [w3421 u32 0 ("New_State")] -> w3277
            tunnel: w3248 -> [w3420 _]
            frame False {
              n1206 = Select(t=u32 1, s=w3420, f=u32 0) -> (s? t:f=w3421:u32)
            }
            frame True {
              n1207 = call-dynamic "Read Channel.vi"("error in (no error)"=w3443, "Acquisition in"=w3444) -> ("error out"=w3427:errorcluster, "Channel.lvclass"=w3430:refnum<class "Channel.lvclass">, "Acquisition out"=w3442:refnum<class "Acquisition.lvclass">)  [unwired: 7 in]
              n1208 = call-dynamic "Write wait_expose.vi"("error in (no error)"=w3427, "wait_expose"=TRUE, "Channel in"=w3430) -> ("error out"=w3426:errorcluster, "Channel out"=w3429:refnum<class "Channel.lvclass">)  [unwired: 7 in]
              n1209 = call-dynamic "Read State Machine.vi"("error in (no error)"=w3426, "Device in"=w3429) -> ("error out"=w3437:errorcluster, "State Machine.lvclass"=w3439:refnum<class "State Machine.lvclass">, "Device out"=w3435:refnum<class "Channel.lvclass">)  [unwired: 7 in]
              n1210 = call "Next State.vi"("error in (no error)"=w3437, "New_State"=40, "State Machine in"=w3439) -> ("error out"=w3432:errorcluster, "State Machine out"=w3433:refnum<class "State Machine.lvclass">)  [unwired: 7 in]
              n1211 = call-dynamic "Write State Machine.vi"("error in (no error)"=w3432, "State Machine.lvclass"=w3433, "Device in"=w3435) -> ("error out"=w3434:errorcluster, "Device out"=w3436:refnum<class "Channel.lvclass">)  [unwired: 7 in]
              n1212 = call-dynamic "Write Channel.vi"("error in (no error)"=w3434, "Channel.lvclass"=w3436, "Acquisition in"=w3442) -> ("error out"=w3440:errorcluster, "Acquisition out"=w3441:refnum<class "Acquisition.lvclass">)  [unwired: 7 in]
            }
          }
          n1213 = call-dynamic "Write AcquisitionA.vi"("error in (no error)"=w3309, "Acquisition.lvclass"=w3311, "S4ACS_GUI in"=w3310) -> ("error out"=w3304:errorcluster, "S4ACS_GUI out"=w3305:refnum<class "S4GUI.lvclass">)  [unwired: 7 in]
          n1214 = call "Read AcquisitionB.vi"("error in (no error)"=w3304, "S4ACS_GUI in"=w3305) -> ("error out"=w3258:errorcluster, "Acquisition.lvclass"=w3260:refnum<class "Acquisition.lvclass">, "S4ACS_GUI out"=w3302:refnum<class "S4GUI.lvclass">)  [unwired: 7 in]
          n1215 = call-dynamic "Read enabled.vi"("error in (no error)"=w3258, "Server in"=w3260) -> ("error out"=w3257:errorcluster, "enabled"=w3247:bool, "Server out"=w3259:refnum<class "Acquisition.lvclass">)  [unwired: 7 in]
          n1216 = call "Read connection.vi"("error in (no error)"=w3257, "Server in"=w3259) -> ("error out"=w3285:errorcluster, "connection"=w3269:bool, "Server out"=w3286:refnum<class "Acquisition.lvclass">)  [unwired: 7 in]
          n1217 = And(x=w3269, y=w3247) -> (x .and. y?=w3270:bool)
          n1218 = case shown="True" w3270 {
            tunnel: w3286 -> [w3400 w3419]
            tunnel: w3285 -> [w3399 w3418]
            tunnel: [w3400 w3416] -> w3303
            tunnel: [w3399 w3415] -> w3301
            tunnel: [w3396 u32 0 ("New_State")] -> w3276
            tunnel: w3247 -> [w3395 _]
            frame False {
              n1219 = Select(t=u32 2, s=w3395, f=u32 0) -> (s? t:f=w3396:u32)
            }
            frame True {
              n1220 = call-dynamic "Read Channel.vi"("error in (no error)"=w3418, "Acquisition in"=w3419) -> ("error out"=w3402:errorcluster, "Channel.lvclass"=w3404:refnum<class "Channel.lvclass">, "Acquisition out"=w3417:refnum<class "Acquisition.lvclass">)  [unwired: 7 in]
              n1221 = call-dynamic "Write wait_expose.vi"("error in (no error)"=w3402, "wait_expose"=TRUE, "Channel in"=w3404) -> ("error out"=w3401:errorcluster, "Channel out"=w3403:refnum<class "Channel.lvclass">)  [unwired: 7 in]
              n1222 = call-dynamic "Read State Machine.vi"("error in (no error)"=w3401, "Device in"=w3403) -> ("error out"=w3412:errorcluster, "State Machine.lvclass"=w3414:refnum<class "State Machine.lvclass">, "Device out"=w3410:refnum<class "Channel.lvclass">)  [unwired: 7 in]
              n1223 = call "Next State.vi"("error in (no error)"=w3412, "New_State"=40, "State Machine in"=w3414) -> ("error out"=w3407:errorcluster, "State Machine out"=w3408:refnum<class "State Machine.lvclass">)  [unwired: 7 in]
              n1224 = call-dynamic "Write State Machine.vi"("error in (no error)"=w3407, "State Machine.lvclass"=w3408, "Device in"=w3410) -> ("error out"=w3409:errorcluster, "Device out"=w3411:refnum<class "Channel.lvclass">)  [unwired: 7 in]
              n1225 = call-dynamic "Write Channel.vi"("error in (no error)"=w3409, "Channel.lvclass"=w3411, "Acquisition in"=w3417) -> ("error out"=w3415:errorcluster, "Acquisition out"=w3416:refnum<class "Acquisition.lvclass">)  [unwired: 7 in]
            }
          }
          n1226 = call "Write AcquisitionB.vi"("error in (no error)"=w3301, "Acquisition.lvclass"=w3303, "S4ACS_GUI in"=w3302) -> ("error out"=w3297:errorcluster, "S4ACS_GUI out"=w3296:refnum<class "S4GUI.lvclass">)  [unwired: 7 in]
          n1227 = call-dynamic "Read AcquisitionC.vi"("error in (no error)"=w3297, "S4ACS_GUI in"=w3296) -> ("error out"=w3254:errorcluster, "Acquisition.lvclass"=w3256:refnum<class "Acquisition.lvclass">, "S4ACS_GUI out"=w3299:refnum<class "S4GUI.lvclass">)  [unwired: 7 in]
          n1228 = call-dynamic "Read enabled.vi"("error in (no error)"=w3254, "Server in"=w3256) -> ("error out"=w3253:errorcluster, "enabled"=w3246:bool, "Server out"=w3255:refnum<class "Acquisition.lvclass">)  [unwired: 7 in]
          n1229 = call "Read connection.vi"("error in (no error)"=w3253, "Server in"=w3255) -> ("error out"=w3283:errorcluster, "connection"=w3266:bool, "Server out"=w3284:refnum<class "Acquisition.lvclass">)  [unwired: 7 in]
          n1230 = And(x=w3266, y=w3246) -> (x .and. y?=w3268:bool)
          n1231 = case shown="True" w3268 {
            tunnel: [w3374 w3388] -> w3300
            tunnel: [w3375 w3387] -> w3298
            tunnel: w3284 -> [w3375 w3385]
            tunnel: w3283 -> [w3374 w3384]
            tunnel: [w3371 u32 0 ("New_State")] -> w3275
            tunnel: w3246 -> [w3370 _]
            frame False {
              n1232 = Select(t=u32 4, s=w3370, f=u32 0) -> (s? t:f=w3371:u32)
            }
            frame True {
              n1233 = call-dynamic "Read Channel.vi"("error in (no error)"=w3384, "Acquisition in"=w3385) -> ("error out"=w3377:errorcluster, "Channel.lvclass"=w3379:refnum<class "Channel.lvclass">, "Acquisition out"=w3386:refnum<class "Acquisition.lvclass">)  [unwired: 7 in]
              n1234 = call-dynamic "Write wait_expose.vi"("error in (no error)"=w3377, "wait_expose"=TRUE, "Channel in"=w3379) -> ("error out"=w3376:errorcluster, "Channel out"=w3378:refnum<class "Channel.lvclass">)  [unwired: 7 in]
              n1235 = call-dynamic "Read State Machine.vi"("error in (no error)"=w3376, "Device in"=w3378) -> ("error out"=w3391:errorcluster, "State Machine.lvclass"=w3389:refnum<class "State Machine.lvclass">, "Device out"=w3393:refnum<class "Channel.lvclass">)  [unwired: 7 in]
              n1236 = call "Next State.vi"("error in (no error)"=w3391, "New_State"=40, "State Machine in"=w3389) -> ("error out"=w3383:errorcluster, "State Machine out"=w3382:refnum<class "State Machine.lvclass">)  [unwired: 7 in]
              n1237 = call-dynamic "Write State Machine.vi"("error in (no error)"=w3383, "State Machine.lvclass"=w3382, "Device in"=w3393) -> ("error out"=w3394:errorcluster, "Device out"=w3392:refnum<class "Channel.lvclass">)  [unwired: 7 in]
              n1238 = call-dynamic "Write Channel.vi"("error in (no error)"=w3394, "Channel.lvclass"=w3392, "Acquisition in"=w3386) -> ("error out"=w3388:errorcluster, "Acquisition out"=w3387:refnum<class "Acquisition.lvclass">)  [unwired: 7 in]
            }
          }
          n1239 = call-dynamic "Write AcquisitionC.vi"("error in (no error)"=w3300, "Acquisition.lvclass"=w3298, "S4ACS_GUI in"=w3299) -> ("error out"=w3294:errorcluster, "S4ACS_GUI out"=w3293:refnum<class "S4GUI.lvclass">)  [unwired: 7 in]
          n1240 = call-dynamic "Read AcquisitionD.vi"("error in (no error)"=w3294, "S4ACS_GUI in"=w3293) -> ("error out"=w3250:errorcluster, "Acquisition.lvclass"=w3252:refnum<class "Acquisition.lvclass">, "S4ACS_GUI out"=w3292:refnum<class "S4GUI.lvclass">)  [unwired: 7 in]
          n1241 = call-dynamic "Read enabled.vi"("error in (no error)"=w3250, "Server in"=w3252) -> ("error out"=w3249:errorcluster, "enabled"=w3245:bool, "Server out"=w3251:refnum<class "Acquisition.lvclass">)  [unwired: 7 in]
          n1242 = call "Read connection.vi"("error in (no error)"=w3249, "Server in"=w3251) -> ("error out"=w3281:errorcluster, "connection"=w3265:bool, "Server out"=w3282:refnum<class "Acquisition.lvclass">)  [unwired: 7 in]
          n1243 = And(x=w3265, y=w3245) -> (x .and. y?=w3267:bool)
          n1244 = case shown="True" w3267 {
            tunnel: w3281 -> [w3349 w3369]
            tunnel: [w3349 w3368] -> w3295
            tunnel: w3282 -> [w3350 w3361]
            tunnel: [w3350 w3359] -> w3291
            tunnel: [w3346 u32 0 ("New_State")] -> w3274
            tunnel: w3245 -> [w3345 _]
            frame False {
              n1245 = Select(t=u32 8, s=w3345, f=u32 0) -> (s? t:f=w3346:u32)
            }
            frame True {
              n1246 = call-dynamic "Read Channel.vi"("error in (no error)"=w3369, "Acquisition in"=w3361) -> ("error out"=w3351:errorcluster, "Channel.lvclass"=w3354:refnum<class "Channel.lvclass">, "Acquisition out"=w3360:refnum<class "Acquisition.lvclass">)  [unwired: 7 in]
              n1247 = call-dynamic "Write wait_expose.vi"("error in (no error)"=w3351, "wait_expose"=TRUE, "Channel in"=w3354) -> ("error out"=w3352:errorcluster, "Channel out"=w3353:refnum<class "Channel.lvclass">)  [unwired: 7 in]
              n1248 = call-dynamic "Read State Machine.vi"("error in (no error)"=w3352, "Device in"=w3353) -> ("error out"=w3365:errorcluster, "State Machine.lvclass"=w3367:refnum<class "State Machine.lvclass">, "Device out"=w3363:refnum<class "Channel.lvclass">)  [unwired: 7 in]
              n1249 = call "Next State.vi"("error in (no error)"=w3365, "New_State"=40, "State Machine in"=w3367) -> ("error out"=w3357:errorcluster, "State Machine out"=w3358:refnum<class "State Machine.lvclass">)  [unwired: 7 in]
              n1250 = call-dynamic "Write State Machine.vi"("error in (no error)"=w3357, "State Machine.lvclass"=w3358, "Device in"=w3363) -> ("error out"=w3362:errorcluster, "Device out"=w3364:refnum<class "Channel.lvclass">)  [unwired: 7 in]
              n1251 = call-dynamic "Write Channel.vi"("error in (no error)"=w3362, "Channel.lvclass"=w3364, "Acquisition in"=w3360) -> ("error out"=w3368:errorcluster, "Acquisition out"=w3359:refnum<class "Acquisition.lvclass">)  [unwired: 7 in]
            }
          }
          n1252 = call-dynamic "Write AcquisitionD.vi"("error in (no error)"=w3295, "Acquisition.lvclass"=w3291, "S4ACS_GUI in"=w3292) -> ("error out"=w3290:errorcluster, "S4ACS_GUI out"=w3289:refnum<class "S4GUI.lvclass">)  [unwired: 7 in]
          n1253 = Compound Arithmetic op=ADD(w3277, w3276, w3275, w3274) -> (w3278:u32)
          n1254 = case shown="0, Default" w3278 {
            tunnel: w3273 -> [w3314 _ _ _ _ _ _ _ _ _ _ _ _ _ _ _]
            tunnel: [w3313 u32 1 ("Obs_state") u32 1 ("Obs_state") u32 1 ("Obs_state") u32 1 ("Obs_state") u32 1 ("Obs_state") u32 1 ("Obs_state") u32 1 ("Obs_state") u32 1 ("Obs_state") u32 1 ("Obs_state") u32 1 ("Obs_state") u32 1 ("Obs_state") u32 1 ("Obs_state") u32 1 ("Obs_state") u32 1 ("Obs_state") u32 1 ("Obs_state")] -> w3279
            tunnel: ["" ("Error Msg") "ERROR: Lost channel 1 connection... - HandleObservationSync.vi state 321" ("Error Msg") "ERROR: Lost channel 2 connection...- HandleObservationSync.vi state 321" ("Error Msg") "ERROR: Lost channels 1 and 2 connection...- HandleObservationSync.vi state 321" ("Error Msg") "ERROR: Lost channel 3 connection...- HandleObservationSync.vi state 321" ("Error Msg") "ERROR: Lost channels 1 and  3 connection...- HandleObservationSync.vi state 321" ("Error Msg") "ERROR:  Lost channels 2 and  3 connection...- HandleObservationSync.vi state 321" ("Error Msg") "ERROR:  Lost channels 1, 2 and  3 connection...- HandleObservationSync.vi state 321" ("Error Msg") "ERROR: Lost channel 4 connection...- HandleObservationSync.vi state 321" ("Error Msg") "ERROR:  Lost channels 1 and 4 connection...- HandleObservationSync.vi state 321" ("Error Msg") "ERROR:  Lost channels 2 and 4 connection...- HandleObservationSync.vi state 321" ("Error Msg") "ERROR: Lost channels 1, 2 and 4 connection...- HandleObservationSync.vi state 321" ("Error Msg") "ERROR: Lost channels 3 and 4 connection...- HandleObservationSync.vi state 321" ("Error Msg") "ERROR: Lost channels 1, 3 and 4 connection...- HandleObservationSync.vi state 321" ("Error Msg") "ERROR: Lost channels 2, 3 and 4 connection...- HandleObservationSync.vi state 321" ("Error Msg") "ERROR: Lost channels 1, 2, 3 and 4 connection...- HandleObservationSync.vi state 321" ("Error Msg")] -> w3280
            frame 0, Default {
              n1255 = Increment(x=w3314) -> (x+1=w3313:u32)
            }
            frame 1 {
            }
            frame 2 {
            }
            frame 3 {
            }
            frame 4 {
            }
            frame 5 {
            }
            frame 6 {
            }
            frame 7 {
            }
            frame 8 {
            }
            frame 9 {
            }
            frame 10 {
            }
            frame 11 {
            }
            frame 12 {
            }
            frame 13 {
            }
            frame 14 {
            }
            frame 15 {
            }
          }
          n1256 = Bundle By Name(cluster=w3289, "Obs_state"=w3279, "Error Msg"=w3280) -> (w3306:refnum<class "S4GUI.lvclass">)
        }
        frame 322 {
          # "Espera terminar o envio de WAIT EXPOSE COMMAND para todos os ACS."
          n1257 = call-dynamic "VerifyAcqIdle.vi"("error in (no error)"=w3446, "S4GUI in"=w3445) -> ("error out"=w3451:errorcluster, "idle"=w3450:bool, "S4GUI out"=w3452:refnum<class "S4GUI.lvclass">)  [unwired: 7 in]
          n1258 = disable-structure shown="Enabled" {
            disable-tunnel: w3448 -> [w3455 _]
            disable-tunnel: [w3454 u32 325] -> w3447
            frame Disabled {
              n1259 = Increment(x=w3455) -> (x+1=w3454:u32)
            }
            frame Enabled {
            }
          }
          n1260 = Select(t=w3447, s=w3450, f=w3448) -> (s? t:f=w3449:u32)
          n1261 = Bundle By Name(cluster=w3452, "Obs_state"=w3449) -> (w3453:refnum<class "S4GUI.lvclass">)
        }
        frame 323 {
          n1262 = call-dynamic "Read AcquisitionA.vi"("error in (no error)"=w3519, "S4ACS_GUI in"=w3520) -> ("error out"=w3474:errorcluster, "Acquisition.lvclass"=w3475:refnum<class "Acquisition.lvclass">, "S4ACS_GUI out"=w3522:refnum<class "S4GUI.lvclass">)  [unwired: 7 in]
          n1263 = call-dynamic "Read enabled.vi"("error in (no error)"=w3474, "Server in"=w3475) -> ("error out"=w3473:errorcluster, "enabled"=w3460:bool, "Server out"=w3476:refnum<class "Acquisition.lvclass">)  [unwired: 7 in]
          n1264 = call "Read connection.vi"("error in (no error)"=w3473, "Server in"=w3476) -> ("error out"=w3499:errorcluster, "connection"=w3483:bool, "Server out"=w3500:refnum<class "Acquisition.lvclass">)  [unwired: 7 in]
          n1265 = And(x=w3483, y=w3460) -> (x .and. y?=w3484:bool)
          n1266 = case shown="True" w3484 {
            tunnel: w3500 -> [w3629 w3645]
            tunnel: w3499 -> [w3628 w3644]
            tunnel: [w3629 w3642] -> w3523
            tunnel: [w3628 w3641] -> w3521
            tunnel: [w3625 u32 0 ("New_State")] -> w3489
            tunnel: w3460 -> [w3624 _]
            frame False {
              n1267 = Select(t=u32 1, s=w3624, f=u32 0) -> (s? t:f=w3625:u32)
            }
            frame True {
              n1268 = call-dynamic "Read Channel.vi"("error in (no error)"=w3644, "Acquisition in"=w3645) -> ("error out"=w3637:errorcluster, "Channel.lvclass"=w3636:refnum<class "Channel.lvclass">, "Acquisition out"=w3643:refnum<class "Acquisition.lvclass">)  [unwired: 7 in]
              n1269 = call-dynamic "Read State Machine.vi"("error in (no error)"=w3637, "Device in"=w3636) -> ("error out"=w3638:errorcluster, "State Machine.lvclass"=w3640:refnum<class "State Machine.lvclass">, "Device out"=w3634:refnum<class "Channel.lvclass">)  [unwired: 7 in]
              n1270 = call "Next State.vi"("error in (no error)"=w3638, "New_State"=50, "State Machine in"=w3640) -> ("error out"=w3631:errorcluster, "State Machine out"=w3632:refnum<class "State Machine.lvclass">)  [unwired: 7 in]
              n1271 = call-dynamic "Write State Machine.vi"("error in (no error)"=w3631, "State Machine.lvclass"=w3632, "Device in"=w3634) -> ("error out"=w3633:errorcluster, "Device out"=w3635:refnum<class "Channel.lvclass">)  [unwired: 7 in]
              n1272 = call-dynamic "Write Channel.vi"("error in (no error)"=w3633, "Channel.lvclass"=w3635, "Acquisition in"=w3643) -> ("error out"=w3641:errorcluster, "Acquisition out"=w3642:refnum<class "Acquisition.lvclass">)  [unwired: 7 in]
            }
          }
          n1273 = call-dynamic "Write AcquisitionA.vi"("error in (no error)"=w3521, "Acquisition.lvclass"=w3523, "S4ACS_GUI in"=w3522) -> ("error out"=w3516:errorcluster, "S4ACS_GUI out"=w3517:refnum<class "S4GUI.lvclass">)  [unwired: 7 in]
          n1274 = call "Read AcquisitionB.vi"("error in (no error)"=w3516, "S4ACS_GUI in"=w3517) -> ("error out"=w3470:errorcluster, "Acquisition.lvclass"=w3472:refnum<class "Acquisition.lvclass">, "S4ACS_GUI out"=w3514:refnum<class "S4GUI.lvclass">)  [unwired: 7 in]
          n1275 = call-dynamic "Read enabled.vi"("error in (no error)"=w3470, "Server in"=w3472) -> ("error out"=w3469:errorcluster, "enabled"=w3459:bool, "Server out"=w3471:refnum<class "Acquisition.lvclass">)  [unwired: 7 in]
